vi "Send SUBSCRIBE.vi"(8 "Subscription Request":T9, 9 "Message Loop Data (in)":T1, 10 "error in (no error)":errorcluster, 11 "WAMP Client in":refnum<class "WAMP Client.lvclass">) -> (1 "Message Loop Data (out)":T1, 2 "error out":errorcluster, 3 "WAMP Client out":refnum<class "WAMP Client.lvclass">)   [LabVIEW 2020, in "wamplv.lvlib" / "WAMP Client.lvclass"]
uses:
  <userlib>/wamplv/WAMP Client/WAMP Client.lvclass
  <userlib>/wamplv/WAMP Client/TypeDef/Message Loop Shift Reg Data.ctl
  <userlib>/wamplv/WAMP Client/TypeDef/REGISTER Request Data.ctl
  <userlib>/wamplv/WAMP Client/TypeDef/REGISTERED or ERROR payload.ctl
  <userlib>/wamplv/WAMP Client/TypeDef/WAMP Error Payload.ctl
  <userlib>/wamplv/WAMP Client/TypeDef/INVOCATION payload.ctl
  <userlib>/wamplv/WAMP Client/TypeDef/Publish Requests Map.ctl
  <userlib>/wamplv/WAMP Client/TypeDef/PUBLISH Request Data.ctl
  <userlib>/wamplv/WAMP Client/TypeDef/PUBLISH Result.ctl
  <userlib>/wamplv/WAMP Client/TypeDef/Endpoint Data.ctl
  <userlib>/wamplv/WAMP Client/TypeDef/CALL Request Map.ctl
  <userlib>/wamplv/WAMP Client/TypeDef/CALL Request Data.ctl
  <userlib>/wamplv/WAMP Client/TypeDef/RESULT Payload.ctl
  <userlib>/wamplv/WAMP Client/TypeDef/SUBSCRIBE Requests Map.ctl
  <userlib>/wamplv/WAMP Client/TypeDef/SUBSCRIBE Request Data.ctl
  <userlib>/wamplv/WAMP Client/TypeDef/Subscribe Result.ctl
  <userlib>/wamplv/WAMP Client/TypeDef/Event Payload.ctl
  <userlib>/wamplv/WAMP Client/TypeDef/Subscriptions Map.ctl
  <userlib>/wamplv/WAMP Client/TypeDef/Subscription Details.ctl
  <userlib>/wamplv/WAMP Client/TypeDef/Unsubscribe Requests Map.ctl
  <userlib>/wamplv/WAMP Client/TypeDef/UNSUBSCRIBE Request Data.ctl
  <userlib>/wamplv/WAMP Client/TypeDef/UNSUBSCRIBE Result.ctl
  <userlib>/wamplv/WAMP Message Codes.ctl
  <userlib>/wamplv/WAMP Client/WAMP Client.lvclass/WAMP Client.ctl
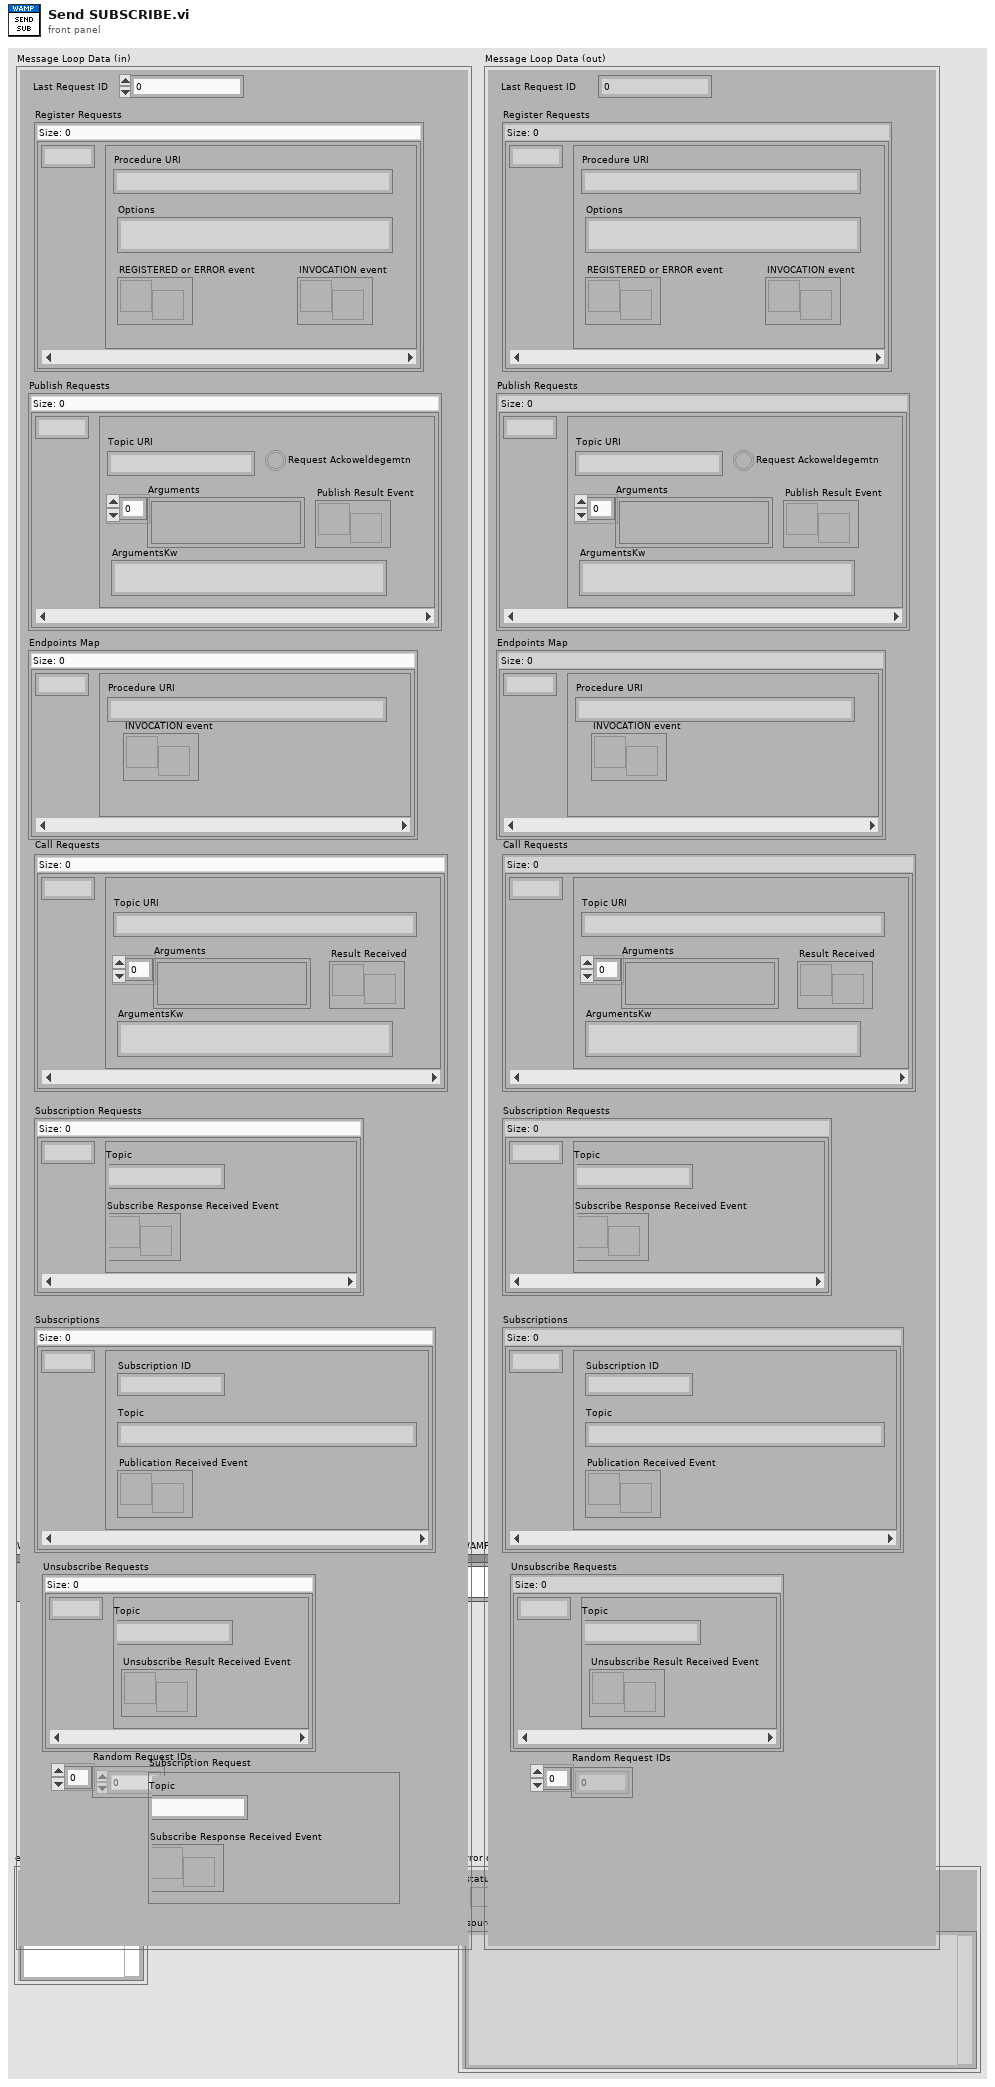
[diagram p1: front panel]
types:
  T1 = typedef "wamplv.lvlib/WAMP Client.lvclass/Message Loop Shift Reg Data.ctl" = cluster{"Last Request ID":u32, "Register Requests":map{u32, T2}, "Publish Requests":T3, "Endpoints Map":map{u32, T5}, "Call Requests":T6, "Subscription Requests":T8, "Subscriptions":T10, "Unsubscribe Requests":T12, "Random Request IDs":u32[]}
  T2 = typedef "wamplv.lvlib/WAMP Client.lvclass/REGISTER Request Data.ctl" = cluster{"Procedure URI":string, "Options":string, "REGISTERED or ERROR event":refnum<user-event>, "INVOCATION event":refnum<user-event>}
  T3 = typedef "wamplv.lvlib/WAMP Client.lvclass/Publish Requests Map.ctl" = map{u32, T4}
  T4 = typedef "wamplv.lvlib/WAMP Client.lvclass/PUBLISH Request Data.ctl" = cluster{"Topic URI":string, "Arguments":variant[], "ArgumentsKw":string, "Publish Result Event":refnum<user-event>, "Request Ackoweldegemtn":bool}
  T5 = typedef "wamplv.lvlib/WAMP Client.lvclass/Endpoint Data.ctl" = cluster{"Procedure URI":string, "INVOCATION event":refnum<user-event>}
  T6 = typedef "wamplv.lvlib/WAMP Client.lvclass/CALL Request Map.ctl" = map{u32, T7}
  T7 = typedef "wamplv.lvlib/WAMP Client.lvclass/CALL Request Data.ctl" = cluster{"Topic URI":string, "Arguments":variant[], "ArgumentsKw":string, "Result Received":refnum<user-event>}
  T8 = typedef "wamplv.lvlib/WAMP Client.lvclass/SUBSCRIBE Requests Map.ctl" = map{u32, T9}
  T9 = typedef "wamplv.lvlib/WAMP Client.lvclass/SUBSCRIBE Request Data.ctl" = cluster{"Topic":string, "Subscribe Response Received Event":refnum<user-event>}
  T10 = typedef "wamplv.lvlib/WAMP Client.lvclass/Subscriptions Map.ctl" = map{u32, T11}
  T11 = typedef "wamplv.lvlib/WAMP Client.lvclass/Subscription Details.ctl" = cluster{"Subscription ID":u32, "Topic":string, "Publication Received Event":refnum<user-event>}
  T12 = typedef "wamplv.lvlib/WAMP Client.lvclass/Unsubscribe Requests Map.ctl" = map{u32, T13}
  T13 = typedef "wamplv.lvlib/WAMP Client.lvclass/UNSUBSCRIBE Request Data.ctl" = cluster{"Topic":string, "Unsubscribe Result Received Event":refnum<user-event>}
  T14 = typedef "wamplv.lvlib/WAMP Client.lvclass/WAMP Message Codes.ctl" = u16
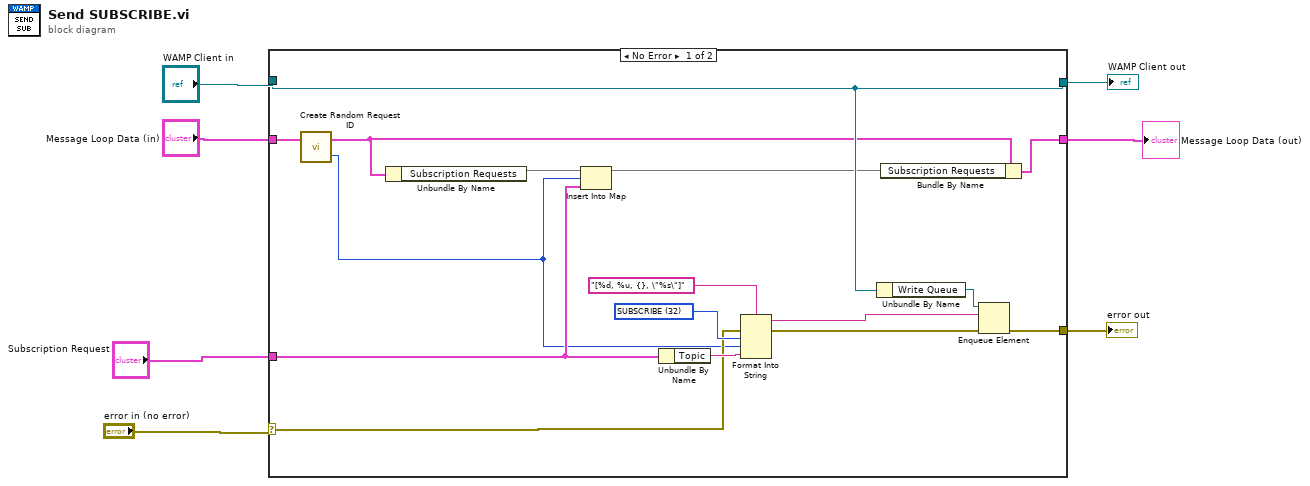
[diagram p0: block diagram]
diagram:
  n1 = case shown="No Error" "error in (no error)" {
    selector: "error in (no error)" -> [w13 w26]
    tunnel: [w16 w26] -> w6
    tunnel: [w19 w25] -> w4
    tunnel: "WAMP Client in" -> [w19 w25]
    tunnel: "Subscription Request" -> [w18 _]
    tunnel: "Message Loop Data (in)" -> [w10 w24]
    tunnel: [w11 w24] -> w1
    frame No Error {
      w20 = T14 32 items=["HELLO"=1, "WELCOME"=2, "ABORT"=3, "GOODBYE"=6, "ERROR"=8, "PUBLISH"=16, "PUBLISHED"=17, "SUBSCRIBE"=32, "SUBSCRIBED"=33, "UNSUBSCRIBE"=34, "UNSUBSCRIBED"=35, "EVENT"=36, "CALL"=48, "RESULT"=59, "REGISTER"=64, "REGISTERED"=65, "UNREGISTER"=66, "UNREGISTERED"=67, "INVOCATION"=68, "YIELD"=70] ("Message Codes")
      n2 = call <userlib>:"Create Random Request ID.vi"("Message Loop Shift Register Data (in)"=w10) -> ("Generated Request ID"=w8:u32, "Message Loop Shift Register Data (out)"=w9:T1)  [unwired: 1 in]
      n3 = Unbundle By Name(w9) -> ("Subscription Requests"=w14:T8)
      n4 = Insert Into Map(map in=w14, key=w8, value=w18) -> (map out=w12:T8)  [unwired: 2 out]
      n5 = Unbundle By Name(w18) -> ("Topic"=w17:string)
      n6 = Format Into String(format string="[%d, %u, {}, \"%s\"]" ("element"), error in=w13, w20, w8, w17) -> (resulting string=w22:string, error out=w23:errorcluster)  [unwired: 1 in]
      n7 = Unbundle By Name(w19) -> ("Write Queue"=w15:refnum<queue>)
      n8 = Bundle By Name(cluster=w9, "Subscription Requests"=w12) -> (w11:T1)
      n9 = Enqueue Element(queue=w15, element=w22, error in (no error)=w23) -> (error out=w16:errorcluster)  [unwired: 1 in, 2 out]
    }
    frame Error {
    }
  }
  "error out" <- w6
  "WAMP Client out" <- w4
  "Message Loop Data (out)" <- w1
